vi "IIC Write Read Bytes.vi"(4 "TimeOutMs":i32, 5 "ReadLen":i32, 6 "WriteLen":i32, 7 "pWriteData":u8[](array[numeric])=array[20480 elements], 9 "SlaveAddr":i16, 10 "IICIndex":i32, 11 "DevIndex":i32) -> (2 "function return":i32, 3 "pReadData":u8[](array[numeric]))   [LabVIEW 2010, in "usb2iic.lvlib"]
doc: "int WINAPI IIC_WriteReadBytes(int DevIndex,int IICIndex,short SlaveAddr,unsigned char *pWriteData,int WriteLen,unsigned char *pReadData,int ReadLen,int TimeOutMs);"
uses:
  usb2iic.lvlib
  USB2XXX.dll
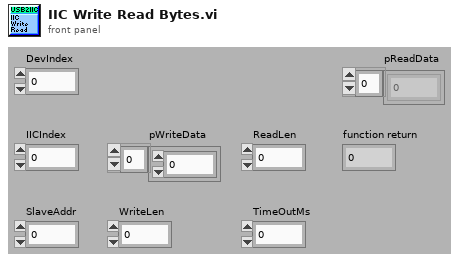
[diagram p1: front panel]
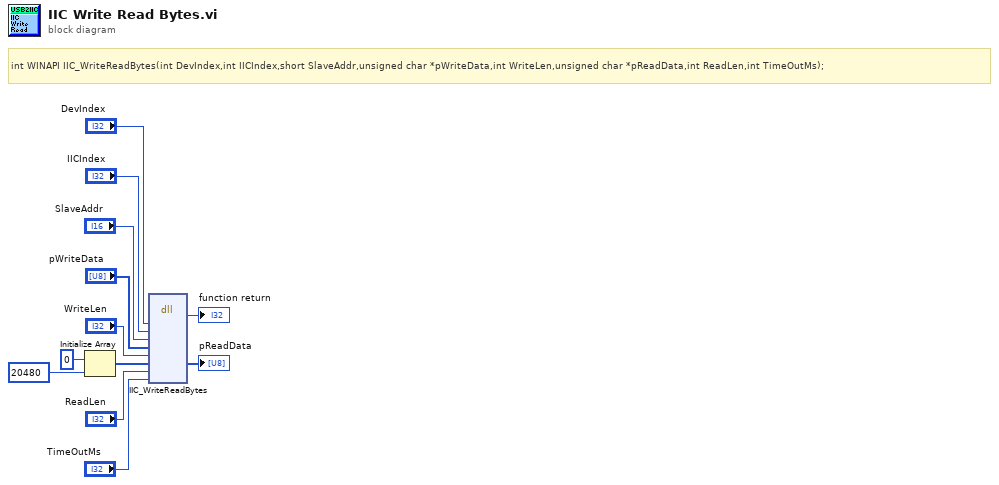
[diagram p0: block diagram]
diagram:
  # "int WINAPI IIC_WriteReadBytes(int DevIndex,int IICIndex,short SlaveAddr,unsigned char *pWriteData,int WriteLen,unsigned char *pReadData,int ReadLen,int TimeOutMs);"
  n1 = Initialize Array(u8 0 ("element"), 20480 ("dimension size")) -> (w6:u8[])
  n2 = dll-call lib="G:/OtherWork/USB2XXX_Example/trunk/Labview/PublicFiles/usb2iic/USB2XXX.*" fn="IIC_WriteReadBytes"("DevIndex"="DevIndex", "IICIndex"="IICIndex", "SlaveAddr"="SlaveAddr", "pWriteData"="pWriteData", "WriteLen"="WriteLen", "pReadData"=w6, "ReadLen"="ReadLen", "TimeOutMs"="TimeOutMs") -> (→"function return":i32, "pReadData"=→"pReadData":u8[])  [unwired: 10 in, 2 out]
